vi "tEST.vi"() -> ()   [LabVIEW 2013, in "Generic Data Logger.lvlib" / "Fluke 2625A (Hydra II).lvlib"]
uses:
  Fluke 2625A (Hydra II).lvlib
panel:
  out "read buffer 2":string
  out "return count 3":u32
  in  "write buffer":string="*OPC?"
  out "String Contains?":bool
  out "return count 2":u32
  out "error out":errorcluster
  out "return count":u32
  out "read buffer":string
  in  "VISA resource name":refnum<visa-resource-name>="COM9"
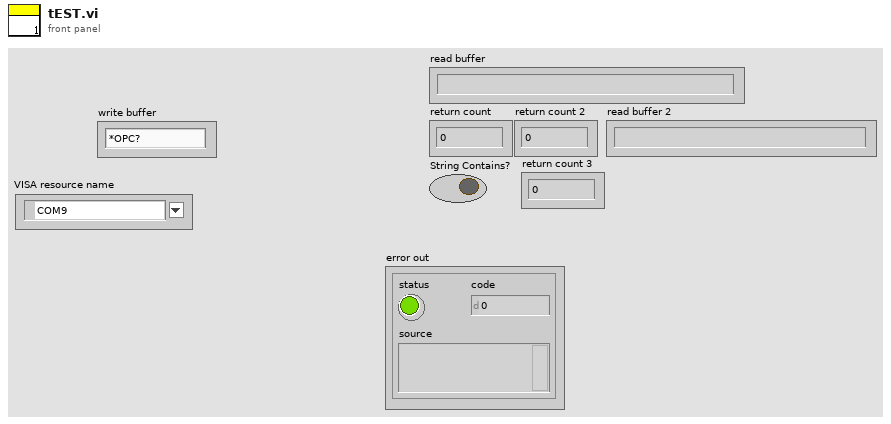
[diagram p1: front panel]
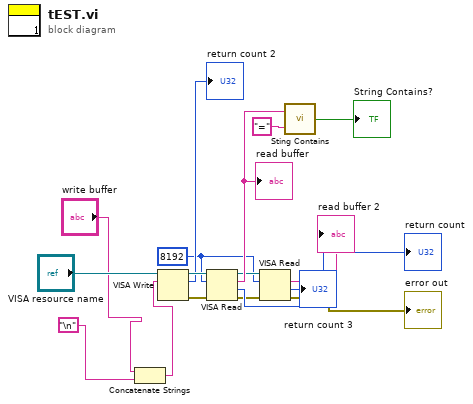
[diagram p0: block diagram]
diagram:
  w7 = u32 8192 ("byte count")
  n1 = Concatenate Strings("write buffer", "\n") -> (w1:string)
  n2 = VISA Write(VISA resource name="VISA resource name", write buffer=w1) -> (VISA resource name out=w16:refnum<visa-resource-name>, return count=→"return count 2":u32, error out=w15:errorcluster)  [unwired: 1 in]
  n3 = VISA Read(VISA resource name=w16, byte count=w7, error in (no error)=w15) -> (VISA resource name out=w9:refnum<visa-resource-name>, read buffer=w12:string, return count=→"return count":u32, error out=w8:errorcluster)
  "read buffer" <- w12
  n4 = VISA Read(VISA resource name=w9, byte count=w7, error in (no error)=w8) -> (read buffer=→"read buffer 2":string, return count=→"return count 3":u32, error out=→"error out":errorcluster)  [unwired: 1 out]
  n5 = call "Sting Contains.vi"("Expression to evaluate"="=", "Input String"=w12) -> ("String Contains?"=→"String Contains?":bool)
